vi "Generic Camera Update Frame Number.vi"(0 "Ref In":T1, 7 "Frame Number":i32, 11 "Error In":errorcluster) -> (4 "Ref Out":T1, 15 "Error Out":errorcluster)   [LabVIEW 2020]
uses:
  <vilib>/vision/Image Controls.llb/IMAQ Image.ctl
  Camera Controls/Camera IMAQ Key Info.ctl
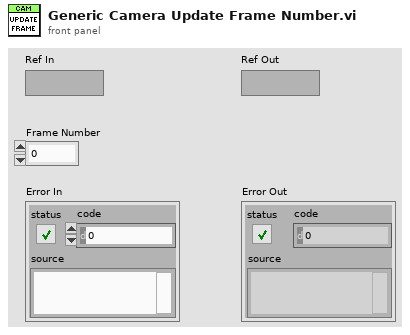
[diagram p1: front panel]
types:
  T1 = typedef "IMAQ Image.ctl" = refnum<image>
  T2 = typedef "Camera IMAQ Key Info.ctl" = cluster{"Frame":u32, "Sensor Height":i32, "Sensor Width":i32, "ROI Height":i32, "ROI Width":i32, "ROI Enable?":bool, "Bit per Pixel":u8}
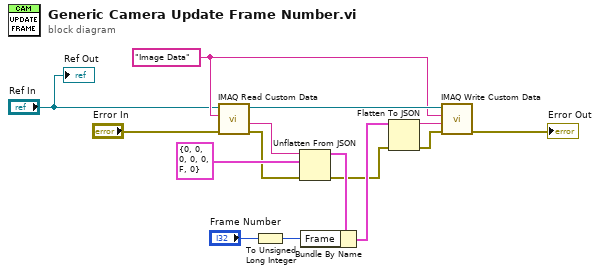
[diagram p0: block diagram]
diagram:
  w8 = "Image Data" ("Key")
  n1 = call "IMAQ Read Custom Data"("error in (no error)"="Error In", "Key"=w8, "Image"="Ref In") -> ("error out"=w7:errorcluster, "Custom Data Out"=w13:string, "Image (duplicate)"=w15:T1)  [unwired: 6 in]
  n2 = To Unsigned Long Integer(number="Frame Number") -> (unsigned 32bit integer=w11:u32)
  n3 = Unflatten From JSON(JSON string=w13, type and defaults=T2 {"Frame"=0, "Sensor Height"=0, "Sensor Width"=0, "ROI Height"=0, "ROI Width"=0, "ROI Enable?"=FALSE, "Bit per Pixel"=0} ("Camera IMAQ Key Info"), error in (no error)=w7) -> (value=w12:T2, error out=w6:errorcluster)  [unwired: 4 in]
  n4 = Bundle By Name(cluster=w12, "Frame"=w11) -> (w10:T2)
  n5 = Flatten To JSON(anything=w10, error in (no error)=w6) -> (JSON string=w9:string, 11:w5:errorcluster)  [unwired: 1 in]
  n6 = call "IMAQ Write Custom Data"("error in (no error)"=w5, "Custom Data In"=w9, "Key"=w8, "Image"=w15) -> ("error out"=→"Error Out":errorcluster)  [unwired: 6 in, 1 out]
  "Ref Out" <- "Ref In"
